vi "post_processing.vi"(8 "error in (no error)":errorcluster, 10 "SSH password":string, 11 "SSH user name":string) -> (0 "error out":errorcluster)   [LabVIEW 2019]
uses:
  ParametersGlobal.vi
panel:
  in  "Date (YYYYMMDD)":string
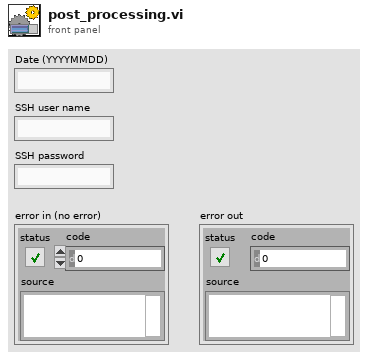
[diagram p1: front panel]
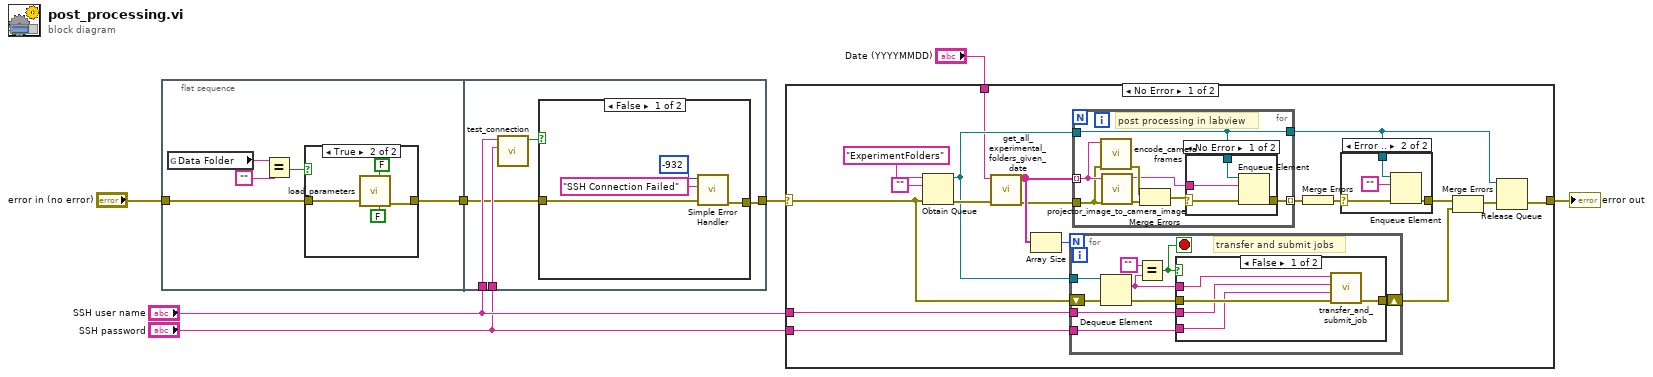
[diagram p0: block diagram]
diagram:
  n1 = flat-sequence {
    tunnel: [w9] -> w5
    tunnel: "error in (no error)" -> [w8]
    tunnel: [w18] -> w6
    tunnel: w5 -> [w19]
    tunnel: "SSH user name" -> [w22]
    tunnel: "SSH password" -> [w21]
    frame #0 {
      n2 = global read "ParametersGlobal.vi" "Data Folder"() -> (w12:string)
      n3 = Equal?(x=w12, y="") -> (x = y?=w10:bool)
      n4 = case shown="True" w10 {
        tunnel: w8 -> [w13 w17]
        tunnel: [w13 w16] -> w9
        frame False {
        }
        frame True {
          n5 = call "load_parameters.vi"("Create Data Folder (T)"=FALSE, "Set Up Projector and Camera (T)"=FALSE, "error in (no error)"=w17) -> ("error out"=w16:errorcluster)  [unwired: 6 in, 2 out]
        }
      }
    }
    frame #1 {
      n6 = call "test_connection.vi"("Username"=w22, "Password"=w21) -> ("Connection Successful"=w20:bool)  [unwired: 7 in]
      n7 = case shown="False" w20 {
        tunnel: w19 -> [w26 w27]
        tunnel: [w25 w27] -> w18
        frame False {
          n8 = call <vilib>:"Simple Error Handler.vi"("error code (no error:0)"=-932, "error source (\" \")"="SSH Connection Failed" ("error source (\" \")"), "error in (no error)"=w26) -> ("error out"=w25:errorcluster)  [unwired: 2 in, 4 out]
        }
        frame True {
        }
      }
    }
  }
  n9 = case shown="No Error" w6 {
    selector: w6 -> [w36 w79]
    tunnel: [w37 w79] -> w7
    tunnel: "SSH password" -> [w34 _]
    tunnel: "SSH user name" -> [w35 _]
    tunnel: "Date (YYYYMMDD)" -> [w28 _]
    frame No Error {
      n10 = Obtain Queue(name (unnamed)="ExperimentFolders", element data type="", error in (no error)=w36) -> (queue out=w40:refnum<queue>, error out=w43:errorcluster)  [unwired: 2 in, 1 out]
      n11 = call "get_all_experimental_folders_given_date.vi"("error in"=w43, "Date (YYYYMMDD)"=w28) -> ("error out"=w33:errorcluster, "Expeirment Folders"=w41:string[])  [unwired: 8 in]
      n12 = Array Size(array=w41) -> (size(s)=w42:i32)
      n13 = for {
        N: w42 -> [_]
        shift-right: [w54] -> w39
        shift-left: w36 -> [w59]
        tunnel: w40 -> [w58]
        tunnel: w35 -> [w52]
        tunnel: w34 -> [w51]
        stop <- w56 stop-if-true
        # "transfer and submit jobs"
        n14 = Dequeue Element(queue=w58, error in (no error)=w59) -> (element=w55:string, error out=w53:errorcluster)  [unwired: 1 in, 2 out]
        n15 = Equal?(x="" ("f"), y=w55) -> (x = y?=w56:bool)
        n16 = case shown="False" w56 {
          tunnel: w55 -> [w64 _]
          tunnel: [w63 w65] -> w54
          tunnel: w53 -> [w62 w65]
          tunnel: w52 -> [w61 _]
          tunnel: w51 -> [w60 _]
          frame False {
            n17 = call "transfer_and_submit_job.vi"("error in (no error)"=w62, "Password"=w60, "Username"=w61, "Experiment Folder"=w64) -> ("error out"=w63:errorcluster)  [unwired: 7 in]
          }
          frame True {
          }
        }
      }
      n18 = for {
        tunnel: w41 -> [w72] mode=indexing
        tunnel: w40 -> [w73]
        tunnel: [w73] -> w29
        tunnel: w33 -> [w66]
        tunnel: [w67] -> w32 mode=indexing
        # "post processing in labview"
        n19 = call "encode_camera_frames.vi"("error in"=w66, "Experiment Folder In"=w72) -> ("Error Out"=w70:errorcluster)  [unwired: 9 in]
        n20 = call "projector_image_to_camera_image.vi"("error in (no error)"=w66, "Experiment Folder in"=w72) -> ("error out"=w71:errorcluster, "Experiment Folder out"=w68:string)  [unwired: 8 in]
        n21 = Merge Errors(w70, w71) -> (w69:errorcluster)
        n22 = case shown="No Error" w69 {
          selector: w69 -> [w75 w78]
          tunnel: [w77 w78] -> w67
          tunnel: w73 -> [w76 _]
          tunnel: w68 -> [w74 _]
          frame No Error {
            n23 = Enqueue Element(queue=w76, element=w74, error in (no error)=w75) -> (error out=w77:errorcluster)  [unwired: 1 in, 2 out]
          }
          frame Error {
          }
        }
      }
      n24 = Merge Errors(w32) -> (w31:errorcluster)
      n25 = case shown="Error .." w31 {
        selector: w31 -> [w46 w50]
        tunnel: [w46 w49] -> w30
        tunnel: w29 -> [_ w48]
        frame No Error {
        }
        frame Error {
          n26 = Enqueue Element(queue=w48, element="" ("f"), error in (no error)=w50) -> (error out=w49:errorcluster)  [unwired: 1 in, 2 out]
        }
      }
      n27 = Merge Errors(w30, w39) -> (w38:errorcluster)
      n28 = Release Queue(queue=w29, error in (no error)=w38) -> (error out=w37:errorcluster)  [unwired: 1 in, 2 out]
    }
    frame Error {
    }
  }
  "error out" <- w7
